vi "References - Get.vi"(8 "error in":errorcluster) -> (0 "error out":errorcluster, 3 "References Out":T1)   [LabVIEW 2024, in "Tester InterComm.lvlib"]
uses:
  Tester InterComm.lvlib
  Type Definitions/Tester References.ctl
  General Actions.ctl
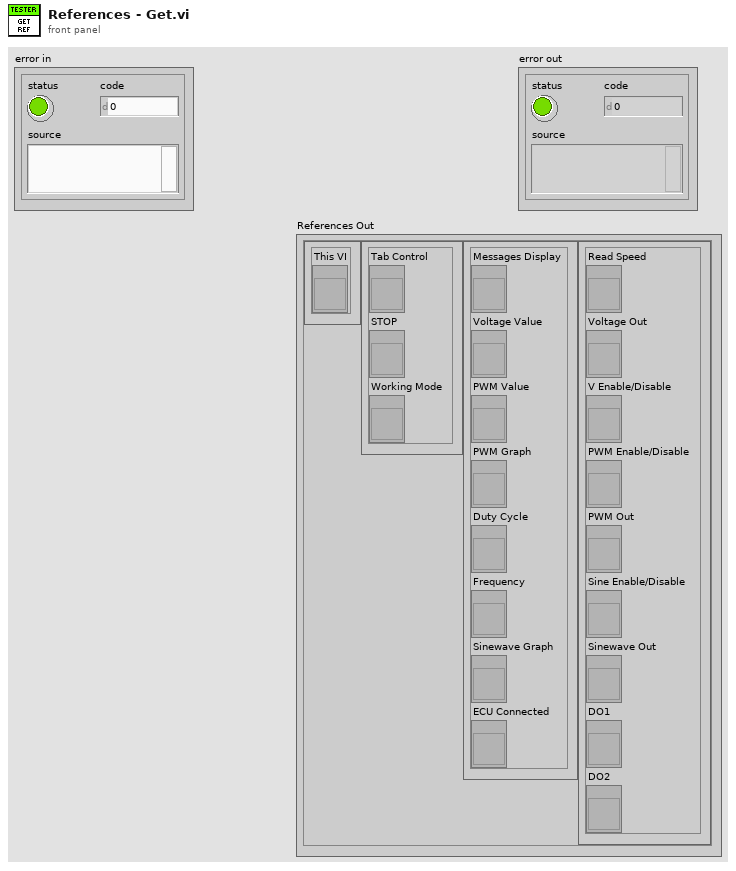
[diagram p1: front panel]
types:
  T1 = typedef "Tester InterComm.lvlib/Tester References.ctl" = cluster{"This VI":cluster{"This VI":refnum<vi>}, "UI Menu":cluster{"Tab Control":refnum<vi>, "STOP":refnum<vi>, "Working Mode":refnum<vi>}, "Indicators":cluster{"Messages Display":refnum<vi>, "Voltage Value":refnum<vi>, "PWM Value":refnum<vi>, "PWM Graph":refnum<vi>, "Duty Cycle":refnum<vi>, "Frequency":refnum<vi>, "Sinewave Graph":refnum<vi>, "ECU Connected":refnum<vi>}, "Controls":cluster{"Read Speed":refnum<vi>, "Voltage Out":refnum<vi>, "V Enable/Disable":refnum<vi>, "PWM Enable/Disable":refnum<vi>, "PWM Out":refnum<vi>, "Sine Enable/Disable":refnum<vi>, "Sinewave Out":refnum<vi>, "DO1":refnum<vi>, "DO2":refnum<vi>}}
  T2 = typedef "Tester InterComm.lvlib/General Actions.ctl" = enum16{"Create", "Get", "Destroy"}
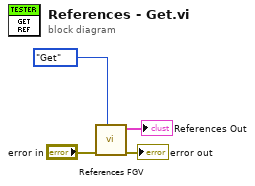
[diagram p0: block diagram]
diagram:
  n1 = call "References FGV.vi"("Ref Action"=General_Actions."Get", "error in"="error in") -> ("error out"=→"error out":errorcluster, "References Out"=→"References Out":T1)  [unwired: 8 in]
